vi "Main.vi"() -> ()   [LabVIEW 2019, in "ModuleD.lvclass"]
uses:
  ModuleD.lvclass
  ModuleB/ModuleStatus.ctl
  ModuleB/ModuleB.lvlib
panel:
  in  "Module Status":T1
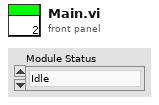
[diagram p1: front panel]
types:
  T1 = typedef "ModuleB.lvlib/ModuleStatus.ctl" = enum16{"Idle", "Running"}
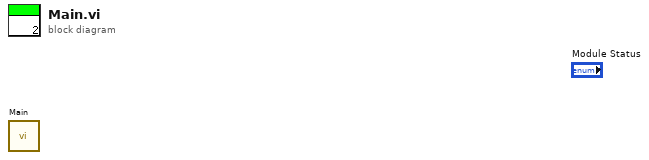
[diagram p0: block diagram]
diagram:
  n1 = call "Main.vi"() -> ()  [unwired: 12 in]
